vi "Exercise 4.1 Webcam Camera.vi"() -> ()   [LabVIEW 2014]
panel:
  out "Output 2":picture
  out "Output":picture
  in  "Image Size":T1(ring)
  in  "camnum":i32
  in  "stop":bool
  out "return type":i32
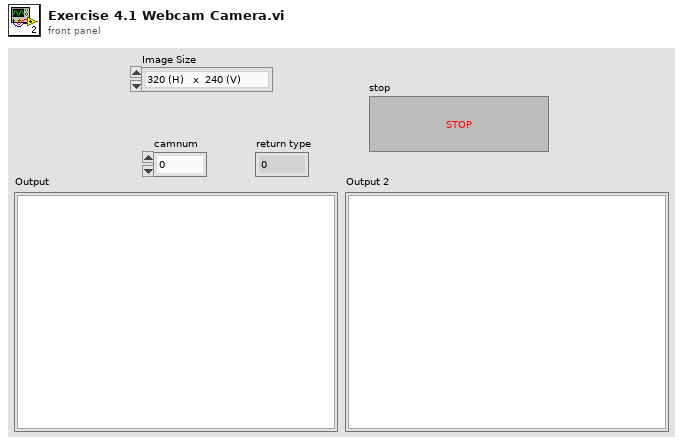
[diagram p1: front panel]
types:
  T1 = enum16{"320 (H)   x  240 (V)", "352(H)    x  288 (V)", "640 (H)   x  480 (V) ", "800 (H)   x  600 (V)", "1024 (H) x  768 (V)", "1280 (H) x  720 (V)", "1280 (H) x 1024 (V)", "1920 (H) x 1080 (V)"}
  T2 = typedef "imagedata.ctl" = cluster{"image type":i32, "image depth":i32, "image":u8[], "mask":u8[], "colors":u32[], "Rectangle":cluster{"left":i16, "top":i16, "right":i16, "bottom":i16}}
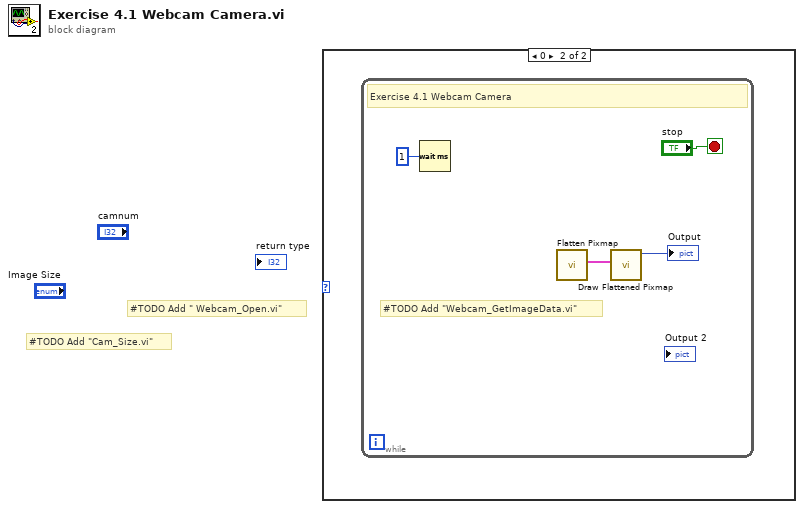
[diagram p0: block diagram]
diagram:
  # "#TODO Add \" Webcam_Open.vi\""
  # "#TODO Add \"Cam_Size.vi\""
  n1 = case shown="0" {
    selector: _ -> [_ _]
    frame -1, Default {
    }
    frame 0 {
      n2 = while {
        stop <- "stop" stop-if-true
        # "#TODO Add \"Webcam_GetImageData.vi\""
        # "Exercise 4.1 Webcam Camera"
        n3 = Wait (ms)(milliseconds to wait=u32 1) -> ()  [unwired: 1 out]
        n4 = call <vilib>:"Flatten Pixmap.vi"() -> ("image data"=w2:T2)  [unwired: 11 in]
        n5 = call <vilib>:"Draw Flattened Pixmap.vi"("image data"=w2) -> ("new picture"=→"Output":picture)  [unwired: 8 in]
      }
    }
  }
